vi "global manueel.vi"() -> ()   [LabVIEW 2019]
panel:
  in  "Boolean manueel":bool
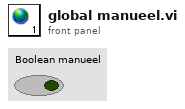
[diagram p1: front panel]
diagram:
